vi "DeliverStim.vi"(5 "Real stim on":bool, 6 "DO error in":errorcluster, 7 "DO task in":refnum<k21>, 8 "AO error in":errorcluster, 9 "AO task in":refnum<k21>) -> (0 "DO error out":errorcluster, 1 "DO task out":refnum<k21>, 2 "AO error out":errorcluster, 3 "AO task out":refnum<k21>, 4 "Time done (s)":dbl format="%_19f")   [LabVIEW 2017]
uses:
  <vilib>/DAQmx/write.llb/DAQmx Write (Digital 1D Bool 1Chan 1Samp).vi
  <vilib>/DAQmx/miscellaneous.llb/DAQmx Fill In Error Info.vi
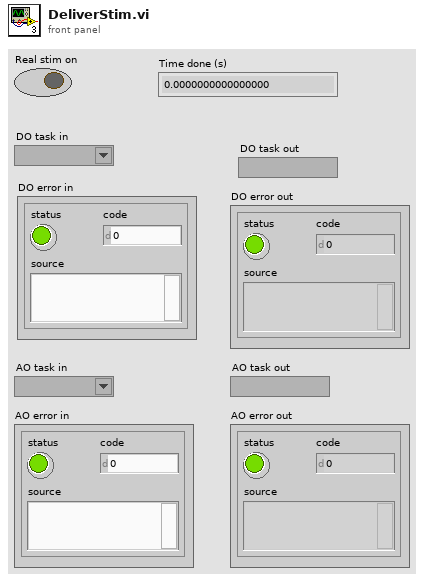
[diagram p1: front panel]
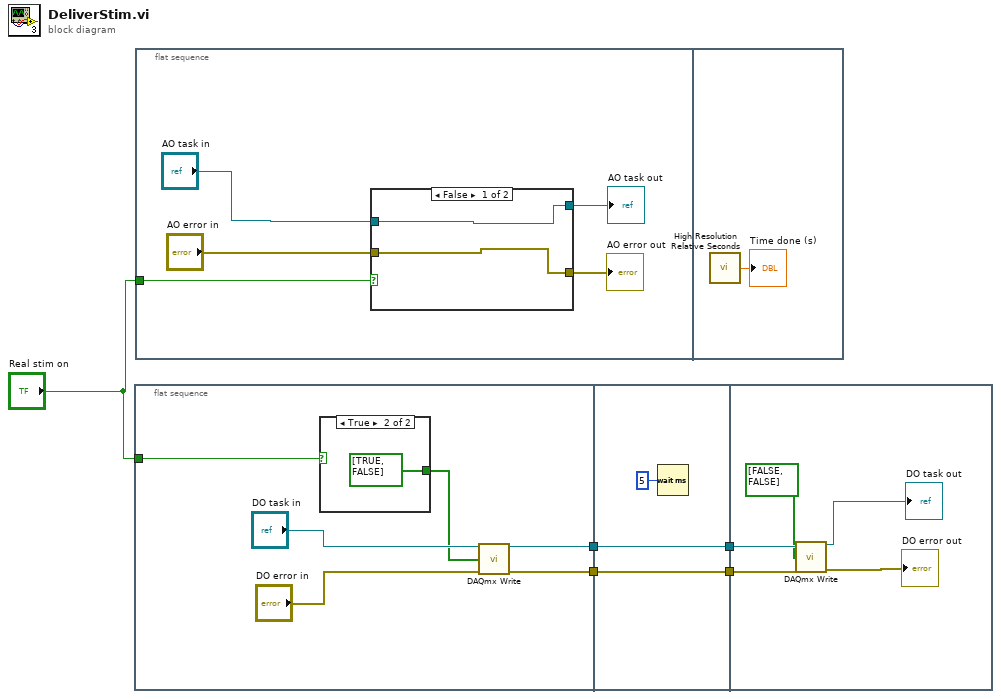
[diagram p0: block diagram]
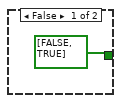
[diagram p2: hidden frame]
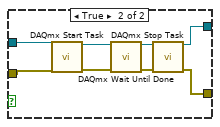
[diagram p3: hidden frame]
diagram:
  n1 = flat-sequence {
    tunnel: "Real stim on" -> [w9]
    tunnel: [w7] -> w4
    tunnel: [w6] -> w3
    tunnel: w4 -> [w16]
    tunnel: w3 -> [w15]
    tunnel: [w16] -> w2
    tunnel: [w15] -> w1
    tunnel: w2 -> [w21]
    tunnel: w1 -> [w20]
    frame #0 {
      n2 = case shown="True" w9 {
        tunnel: [bool[] [FALSE, TRUE] ("data") bool[] [TRUE, FALSE] ("data")] -> w8
        frame False {
        }
        frame True {
        }
      }
      n3 = call-poly <vilib>:"DAQmx Write.vi"("task/channels in"="DO task in", "data"=w8, "error in"="DO error in") -> ("task out"=w7:refnum<k21>, "error out"=w6:errorcluster)  [unwired: 10 in, 1 out]
    }
    frame #1 {
      n4 = Wait (ms)(milliseconds to wait=u32 5) -> ()  [unwired: 1 out]
    }
    frame #2 {
      n5 = call-poly <vilib>:"DAQmx Write.vi"("task/channels in"=w21, "data"=bool[] [FALSE, FALSE], "error in"=w20) -> ("task out"=→"DO task out":refnum<k21>, "error out"=→"DO error out":errorcluster)  [unwired: 10 in, 1 out]
    }
  }
  n6 = flat-sequence {
    tunnel: "Real stim on" -> [w22]
    frame #0 {
      n7 = case shown="False" w22 {
        tunnel: "AO error in" -> [w27 w36]
        tunnel: "AO task in" -> [w28 w35]
        tunnel: [w28 w30] -> w24
        tunnel: [w27 w29] -> w23
        frame False {
        }
        frame True {
          n8 = call <vilib>:"DAQmx Start Task.vi"("task/channels in"=w35, "error in"=w36) -> ("task out"=w32:refnum<k21>, "error out"=w31:errorcluster)  [unwired: 12 in]
          n9 = call <vilib>:"DAQmx Wait Until Done.vi"("task/channels in"=w32, "error in"=w31) -> ("task out"=w34:refnum<k21>, "error out"=w33:errorcluster)  [unwired: 12 in]
          n10 = call <vilib>:"DAQmx Stop Task.vi"("task/channels in"=w34, "error in"=w33) -> ("task out"=w30:refnum<k21>, "error out"=w29:errorcluster)  [unwired: 12 in]
        }
      }
      "AO error out" <- w23
      "AO task out" <- w24
    }
    frame #1 {
      n11 = call <vilib>:"High Resolution Relative Seconds.vi"() -> ("relative seconds"=→"Time done (s)":dbl)
    }
  }
